vi "R1NOControl.vi"(8 "error constant":errorcluster, 11 "LabVIEW Web Service":refnum<class "Web Service.lvclass">) -> (0 "error (out)":errorcluster)   [LabVIEW 2016]
uses:
  <vilib>/wsapi/Web Service.lvclass
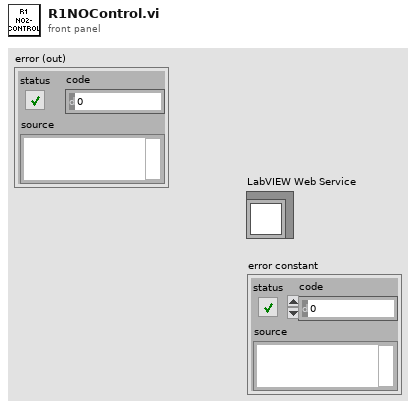
[diagram p1: front panel]
types:
  T1 = cluster{"Set Point, mg/L":dbl, "Tolerance, mg/L":dbl, "N2 Valve Gain":dbl, "Air Valve Gain":dbl}
  T2 = cluster{"Media Pump":bool, "Water Pump":bool, "Effluent Pump":bool, "Release Valve":bool, "Gas Pump":bool}
  T3 = cluster{"Signal, mA":dbl, "Value, UNITS HERE":dbl}
  T4 = cluster{"Nitrite Set Point, mgN/L":dbl, "Check Every X seconds":dbl, "DO Set Point Low, mg/L":dbl, "DO Set Point High, mg/L":dbl}
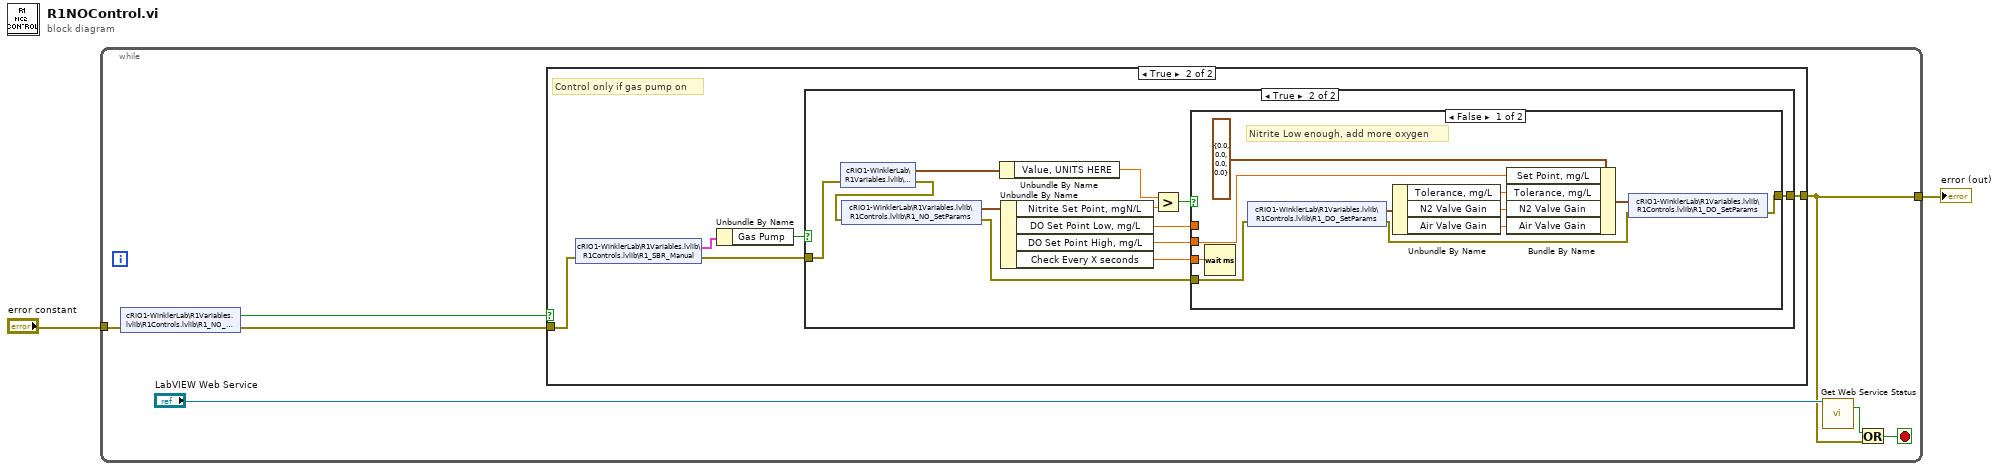
[diagram p0: block diagram]
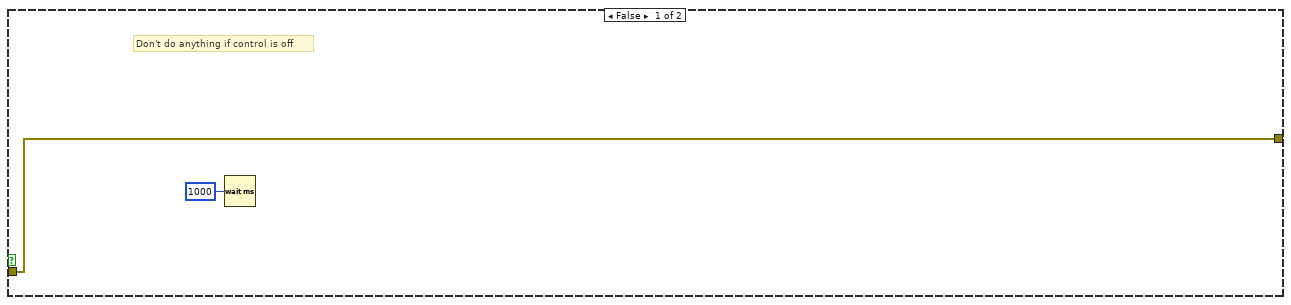
[diagram p2: hidden frame]
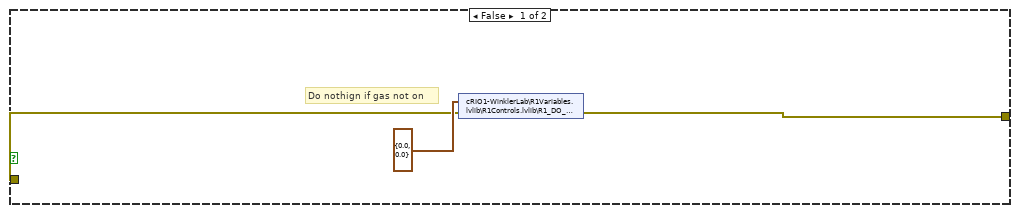
[diagram p3: hidden frame]
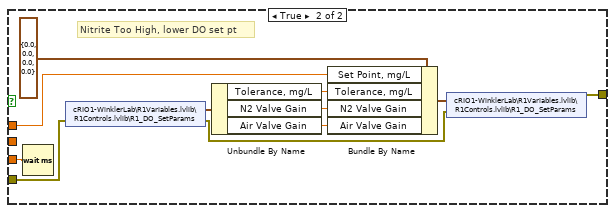
[diagram p4: hidden frame]
diagram:
  n1 = while {
    tunnel: "error constant" -> [w6]
    tunnel: [w3] -> w1
    stop <- w7 stop-if-true
    n2 = shared-variable "cRIO1-WinklerLab\\R1Variables.lvlib\\R1Controls.lvlib\\R1_NO_Switch"(error in=w6) -> (w5:bool, error out=w4:errorcluster)
    n3 = case shown="True" w5 {
      tunnel: w4 -> [w10 w13]
      tunnel: [w10 w12] -> w3
      frame False {
        # "Don't do anything if control is off"
        n4 = Wait (ms)(milliseconds to wait=u32 1000) -> ()  [unwired: 1 out]
      }
      frame True {
        # "Control only if gas pump on"
        n5 = shared-variable "cRIO1-WinklerLab\\R1Variables.lvlib\\R1Controls.lvlib\\R1_SBR_Manual"(error in=w13) -> (w15:T2, error out=w14:errorcluster)
        n6 = Unbundle By Name(w15) -> ("Gas Pump"=w16:bool)
        n7 = case shown="True" w16 {
          tunnel: w14 -> [w18 w30]
          tunnel: [w17 w31] -> w12
          frame False {
            # "Do nothign if gas not on"
            n8 = shared-variable "cRIO1-WinklerLab\\R1Variables.lvlib\\R1Controls.lvlib\\R1_DO_Manual"(cluster{"Air MFC":dbl, "N2 MFC":dbl} {"Air MFC"=0.0, "N2 MFC"=0.0} ("R1DOManual"), error in=w18) -> (error out=w17:errorcluster)
          }
          frame True {
            n9 = shared-variable "cRIO1-WinklerLab\\R1Variables.lvlib\\R1Signals.lvlib\\R1NO"(error in=w30) -> (w29:T3, error out=w28:errorcluster)
            n10 = shared-variable "cRIO1-WinklerLab\\R1Variables.lvlib\\R1Controls.lvlib\\R1_NO_SetParams"(error in=w28) -> (w27:T4, error out=w23:errorcluster)
            n11 = Unbundle By Name(w29) -> ("Value, UNITS HERE"=w26:dbl)
            n12 = Unbundle By Name(w27) -> ("Nitrite Set Point, mgN/L"=w25:dbl, "DO Set Point Low, mg/L"=w21:dbl, "DO Set Point High, mg/L"=w20:dbl, "Check Every X seconds"=w22:dbl)
            n13 = Greater?(x=w26, y=w25) -> (0:w24:bool)
            n14 = case shown="False" w24 {
              tunnel: [w32 w46] -> w31
              tunnel: w23 -> [w35 w48]
              tunnel: w22 -> [w34 w44]
              tunnel: w21 -> [_ w43]
              tunnel: w20 -> [w33 _]
              frame False {
                # "Nitrite Low enough, add more oxygen"
                n15 = Wait (ms)(milliseconds to wait=w34) -> ()  [unwired: 1 out]
                n16 = shared-variable "cRIO1-WinklerLab\\R1Variables.lvlib\\R1Controls.lvlib\\R1_DO_SetParams"(error in=w35) -> (w41:T1, error out=w37:errorcluster)
                n17 = Unbundle By Name(w41) -> ("Tolerance, mg/L"=w38:dbl, "N2 Valve Gain"=w39:dbl, "Air Valve Gain"=w40:dbl)
                n18 = Bundle By Name(cluster=T1 {"Set Point, mg/L"=0.0, "Tolerance, mg/L"=0.0, "N2 Valve Gain"=0.0, "Air Valve Gain"=0.0} ("R1_DO_SetParams"), "Set Point, mg/L"=w33, "Tolerance, mg/L"=w38, "N2 Valve Gain"=w39, "Air Valve Gain"=w40) -> (w36:T1)
                n19 = shared-variable "cRIO1-WinklerLab\\R1Variables.lvlib\\R1Controls.lvlib\\R1_DO_SetParams"(w36, error in=w37) -> (error out=w32:errorcluster)
              }
              frame True {
                # "Nitrite Too High, lower DO set pt"
                n20 = Wait (ms)(milliseconds to wait=w44) -> ()  [unwired: 1 out]
                n21 = shared-variable "cRIO1-WinklerLab\\R1Variables.lvlib\\R1Controls.lvlib\\R1_DO_SetParams"(error in=w48) -> (w52:T1, error out=w47:errorcluster)
                n22 = Unbundle By Name(w52) -> ("Tolerance, mg/L"=w49:dbl, "N2 Valve Gain"=w50:dbl, "Air Valve Gain"=w51:dbl)
                n23 = Bundle By Name(cluster=T1 {"Set Point, mg/L"=0.0, "Tolerance, mg/L"=0.0, "N2 Valve Gain"=0.0, "Air Valve Gain"=0.0} ("R1_DO_SetParams"), "Set Point, mg/L"=w43, "Tolerance, mg/L"=w49, "N2 Valve Gain"=w50, "Air Valve Gain"=w51) -> (w45:T1)
                n24 = shared-variable "cRIO1-WinklerLab\\R1Variables.lvlib\\R1Controls.lvlib\\R1_DO_SetParams"(w45, error in=w47) -> (error out=w46:errorcluster)
              }
            }
          }
        }
      }
    }
    n25 = call <vilib>:"Get Web Service Status.vi"("LabVIEW Web Service"="LabVIEW Web Service") -> ("service stopping?"=w9:bool)  [unwired: 12 in, 2 out]
    n26 = Or(x=w9, y=w3) -> (x .or. y?=w7:bool)
  }
  "error (out)" <- w1
